vi "Test Assert Equal (Float).vi"(8 "error in (no error)":errorcluster) -> (0 "error out":errorcluster)   [LabVIEW 2009]
uses:
  classes/Assert/Assert.lvclass
  classes/Test/Test.lvclass
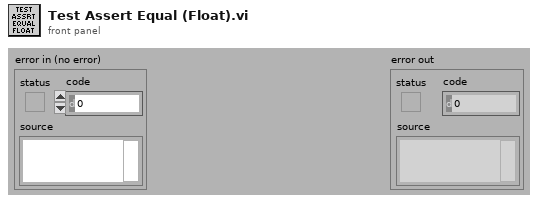
[diagram p1: front panel]
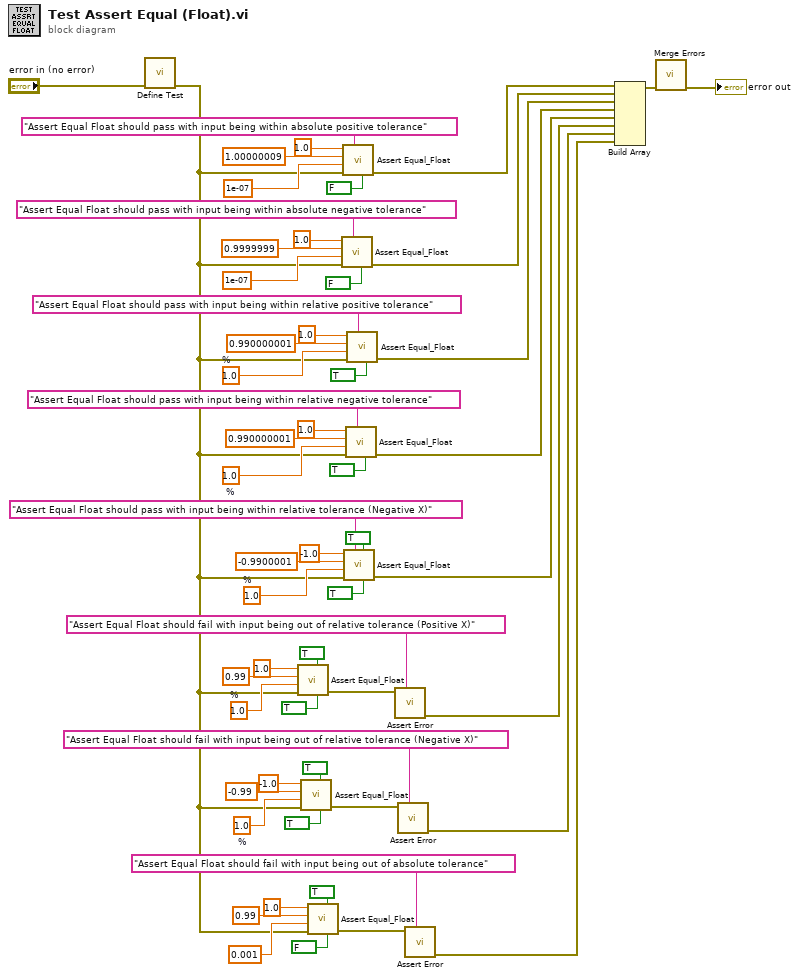
[diagram p0: block diagram]
diagram:
  w7 = 1.0  # %
  w15 = 1.0  # %
  w28 = 1.0  # %
  w35 = 1.0  # %
  w40 = 1.0  # %
  n1 = call "Define Test.vi"("error in (no error)"="error in (no error)") -> ("error out"=w1:errorcluster)  [unwired: 10 in]
  n2 = call "Assert Equal_Float.vi"("Use Percentage of X (F)"=TRUE, "Assert Only? (F)"=TRUE, "error in (no error)"=w1, "Tolerance"=w28, "Y"=0.99, "X"=1.0) -> ("error out"=w26:errorcluster)  [unwired: 5 in]
  n3 = call "Assert Equal_Float.vi"("Use Percentage of X (F)"=TRUE, "Assert Only? (F)"=TRUE, "error in (no error)"=w1, "Tolerance"=w7, "Y"=-0.99, "X"=-1.0) -> ("error out"=w9:errorcluster)  [unwired: 5 in]
  n4 = call "Assert Equal_Float.vi"("Use Percentage of X (F)"=FALSE, "Assert Only? (F)"=TRUE, "error in (no error)"=w1, "Tolerance"=0.001, "Y"=0.99, "X"=1.0) -> ("error out"=w24:errorcluster)  [unwired: 5 in]
  n5 = call "Assert Equal_Float.vi"("Use Percentage of X (F)"=FALSE, "Label"="Assert Equal Float should pass with input being within absolute negative tolerance", "error in (no error)"=w1, "Tolerance"=1e-07, "Y"=0.9999999, "X"=1.0) -> ("error out"=w45:errorcluster)  [unwired: 5 in]
  n6 = call "Assert Equal_Float.vi"("Use Percentage of X (F)"=FALSE, "Label"="Assert Equal Float should pass with input being within absolute positive tolerance", "error in (no error)"=w1, "Tolerance"=1e-07, "Y"=1.00000009, "X"=1.0) -> ("error out"=w55:errorcluster)  [unwired: 5 in]
  n7 = call "Assert Equal_Float.vi"("Use Percentage of X (F)"=TRUE, "Assert Only? (F)"=TRUE, "Label"="Assert Equal Float should pass with input being within relative tolerance (Negative X)", "error in (no error)"=w1, "Tolerance"=w15, "Y"=-0.9900001, "X"=-1.0) -> ("error out"=w10:errorcluster)  [unwired: 4 in]
  n8 = call "Assert Equal_Float.vi"("Use Percentage of X (F)"=TRUE, "Label"="Assert Equal Float should pass with input being within relative negative tolerance", "error in (no error)"=w1, "Tolerance"=w35, "Y"=0.990000001, "X"=1.0) -> ("error out"=w33:errorcluster)  [unwired: 5 in]
  n9 = call "Assert Equal_Float.vi"("Use Percentage of X (F)"=TRUE, "Label"="Assert Equal Float should pass with input being within relative positive tolerance", "error in (no error)"=w1, "Tolerance"=w40, "Y"=0.990000001, "X"=1.0) -> ("error out"=w34:errorcluster)  [unwired: 5 in]
  n10 = call "Assert Error.vi"("Label"="Assert Equal Float should fail with input being out of relative tolerance (Positive X)", "Error?"=w26) -> ("error out"=w25:errorcluster)  [unwired: 9 in]
  n11 = call "Assert Error.vi"("Label"="Assert Equal Float should fail with input being out of relative tolerance (Negative X)", "Error?"=w9) -> ("error out"=w2:errorcluster)  [unwired: 9 in]
  n12 = call "Assert Error.vi"("Label"="Assert Equal Float should fail with input being out of absolute tolerance", "Error?"=w24) -> ("error out"=w17:errorcluster)  [unwired: 9 in]
  n13 = Build Array(w55, w45, w34, w33, w10, w25, w2, w17) -> (w57:errorcluster[])
  n14 = call <vilib>:"Merge Errors.vi"("error array in"=w57) -> ("error out"=→"error out":errorcluster)  [unwired: 6 in]
